vi "BRig_dataBlock_nWrong.vi"() -> (2 "output_nWrong":i32)   [LabVIEW 2014]
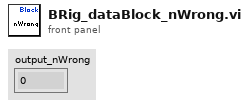
[diagram p1: front panel]
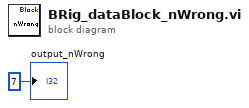
[diagram p0: block diagram]
diagram:
  "output_nWrong" <- 7 ("output_iBlock")
